vi "Go to Voice.vi"(8 "error in (no error)":errorcluster, 11 "CommonState in":refnum<class "CoordinatorState.lvclass">) -> (0 "error out":errorcluster, 3 "CommonState out":refnum<class "State Actor.lvclass">)   [LabVIEW 2014, in "States.lvlib" / "CoordinatorState.lvclass"]
doc: "This method defines the transition from any state to the Running state."
uses:
  CoordinatorState.lvclass
  <vilib>/NI/Actors/State Actor/State Actor/State Actor.lvclass
  Running/Voice.lvclass
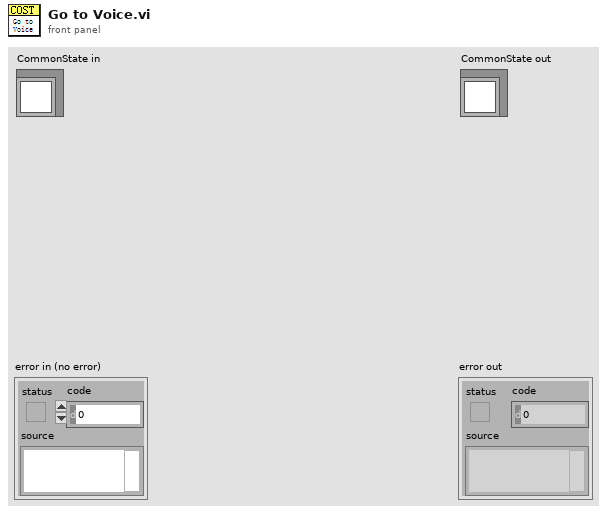
[diagram p1: front panel]
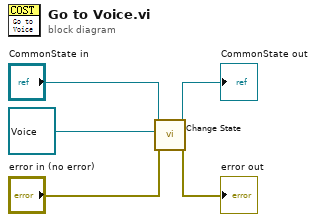
[diagram p0: block diagram]
diagram:
  n1 = call <vilib>:"Change State.vi"("error in (no error)"="error in (no error)", "New State in"=refnum<class "Voice.lvclass"> refnum ("Process States.lvlib:Running.lvclass"), "State in"="CommonState in") -> ("error out"=→"error out":errorcluster, "State out"=→"CommonState out":refnum<class "State Actor.lvclass">)  [unwired: 7 in]
